vi "TCP IP Read Data 5U.vi"(5 "No of data regiter read":i32=4, 7 "Start Address":i32=4, 8 "error in":errorcluster, 10 "Data Rigister/Memory":enum16{"Data Register D", "Intiger M"}(ring), 11 "connection ID":refnum<k5>) -> (0 "error out":errorcluster, 2 "RAw Data":string, 3 "connection ID Out":refnum<k5>)   [LabVIEW 2024]
panel:
  out "s? t:f":string
  out "hex integer string":string
  out "bytes to read":i32
  out "Start Address":string="1028"
  out "length":i32
  out "data out":string
  in  "milliseconds to wait":u32=100
  # "500000FF03FF000018001004010000M*0010000002"
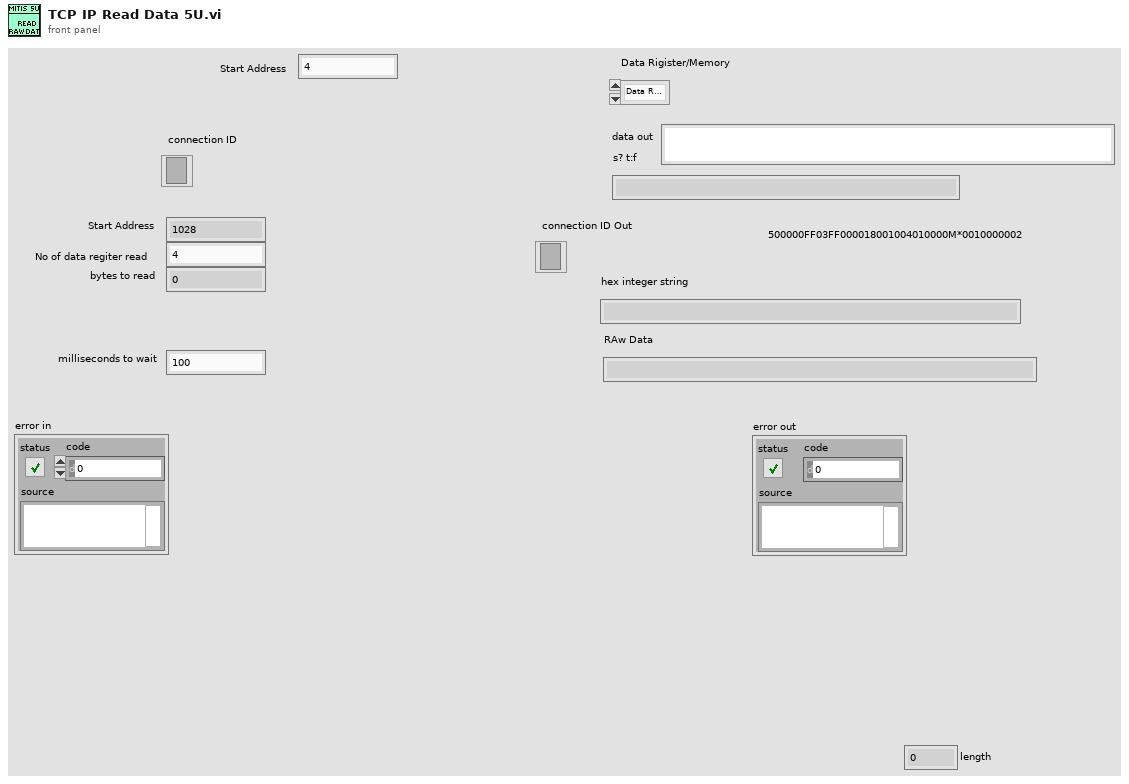
[diagram p1: front panel]
types:
  T1 = enum16{"Standard", "Buffered", "CRLF", "Immediate"}
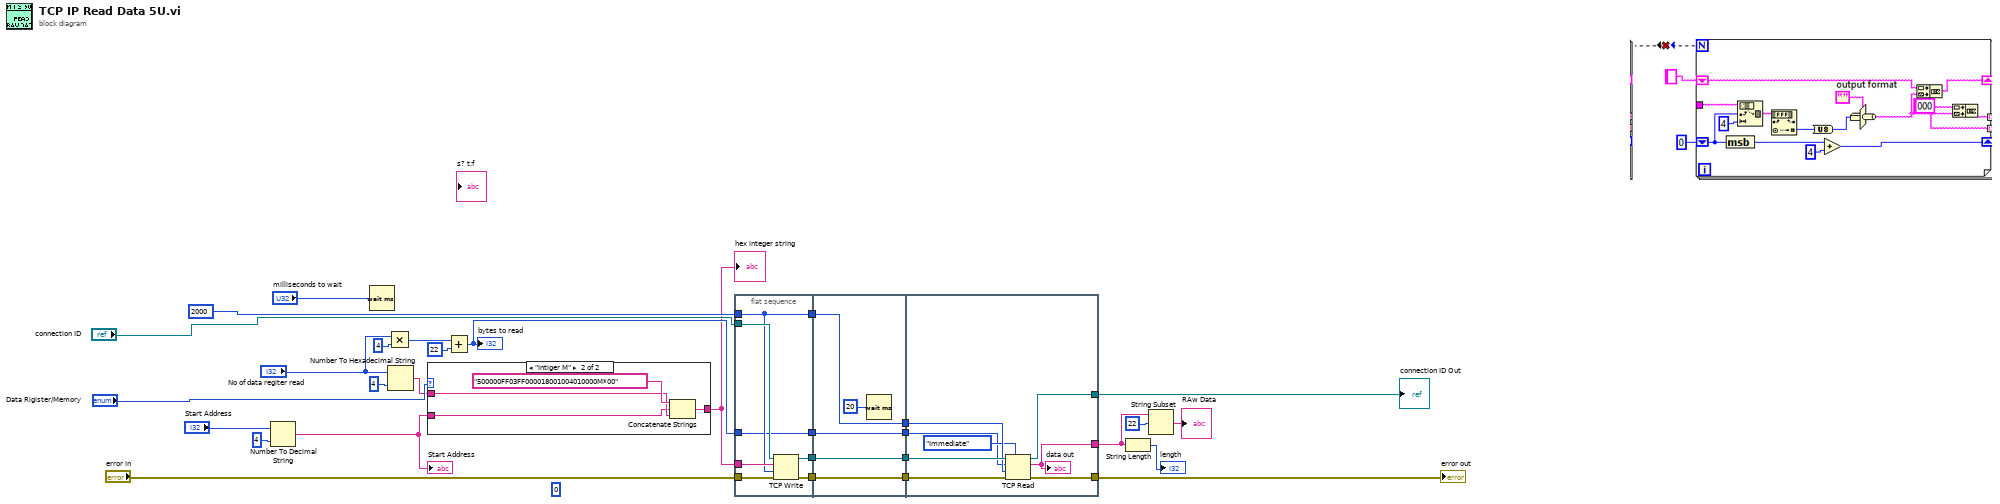
[diagram p0: block diagram]
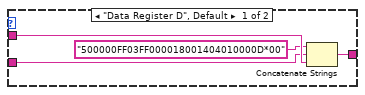
[diagram p2: hidden frame]
diagram:
  (unwired) 0 ("length (rest)")
  n1 = Number To Decimal String(number="Start Address", width (-)=i16 4) -> (decimal integer string=w3:string)
  "Start Address" <- w3
  n2 = Wait (ms)(milliseconds to wait="milliseconds to wait") -> ()  [unwired: 1 out]
  n3 = Multiply(x="No of data regiter read", y=4) -> (x*y=w13:i32)
  n4 = Number To Hexadecimal String(1:i16 4 ("width (-)"), 2:"No of data regiter read") -> (0:w10:string)
  n5 = case shown="\"Data Register D\", Default" "Data Rigister/Memory" {
    tunnel: w10 -> [w34 w37]
    tunnel: [w31 w36] -> w2
    tunnel: w3 -> [w32 w35]
    frame "Data Register D", Default {
      n6 = Concatenate Strings("500000FF03FF000018001404010000D*00", w32, w34) -> (w31:string)
    }
    frame "Intiger M" {
      n7 = Concatenate Strings("500000FF03FF000018001004010000M*00" ("Frame to Read M100 to M107 from FX5U"), w35, w37) -> (w36:string)
    }
  }
  "hex integer string" <- w2
  n8 = Add(x=w13, y=22) -> (x+y=w7:i32)
  "bytes to read" <- w7
  n9 = flat-sequence {
    tunnel: w2 -> [w43]
    tunnel: "error in" -> [w44]
    tunnel: "connection ID" -> [w45]
    tunnel: 2000 ("timeout ms  2") -> [w40]
    tunnel: [w42] -> w24
    tunnel: [w41] -> w23
    tunnel: [w40] -> w22
    tunnel: w7 -> [w39]
    tunnel: [w39] -> w21
    tunnel: [w50] -> w20
    tunnel: w24 -> [w50]
    tunnel: [w49] -> w19
    tunnel: w23 -> [w49]
    tunnel: [w47] -> w18
    tunnel: w22 -> [w47]
    tunnel: [w46] -> w17
    tunnel: w21 -> [w46]
    tunnel: [w58] -> w9
    tunnel: w20 -> [w57]
    tunnel: w19 -> [w56]
    tunnel: w18 -> [w55]
    tunnel: [w53] -> w25
    tunnel: [w52] -> w26
    tunnel: w17 -> [w51]
    frame #0 {
      n10 = TCP Write(connection ID=w45, data in=w43, error in (no error)=w44, 9:w40) -> (connection ID out=w42:refnum<k5>, error out=w41:errorcluster)  [unwired: 1 out]
    }
    frame #1 {
      n11 = Wait (ms)(milliseconds to wait=u32 20) -> ()  [unwired: 1 out]
    }
    frame #2 {
      n12 = TCP Read(connection ID=w57, bytes to read=w51, error in (no error)=w56, 7:T1."Immediate" ("mode (standard)"), 9:w55) -> (connection ID out=w53:refnum<k5>, data out=w58:string, error out=w52:errorcluster)
      "data out" <- w58
    }
  }
  n13 = String Length(string=w9) -> (length=→"length":i32)
  n14 = String Subset(string=w9, offset (0)=22) -> (substring=→"RAw Data":string)  [unwired: 1 in]
  "error out" <- w26
  "connection ID Out" <- w25
